vi "Find Class Ancestry.vi"(8 "error in (no error)":errorcluster, 11 "reference in":refnum<vi>) -> (0 "error out":errorcluster, 3 "Class Ancestry":path[](array[path]))   [LabVIEW 2020, in "Test Suite Factory.lvclass"]
uses:
  Test Suite Factory.lvclass
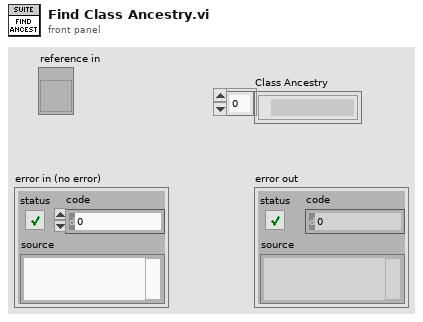
[diagram p1: front panel]
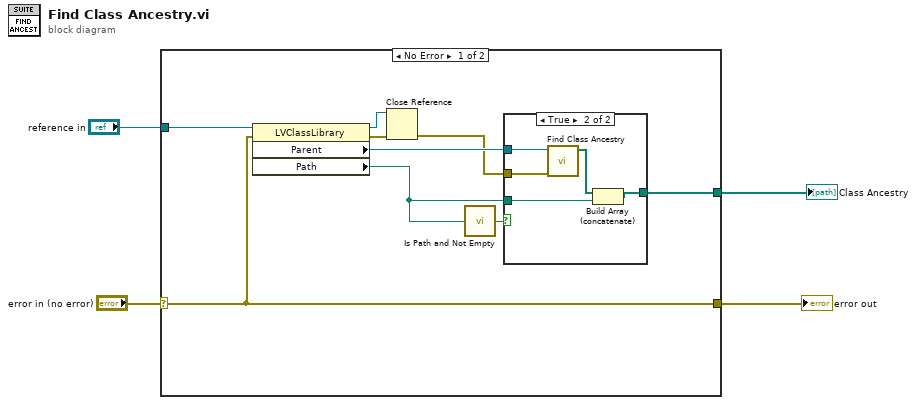
[diagram p0: block diagram]
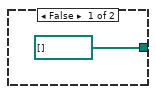
[diagram p2: hidden frame]
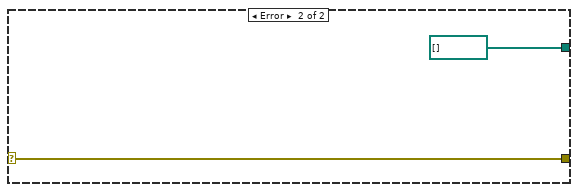
[diagram p3: hidden frame]
diagram:
  n1 = case shown="No Error" "error in (no error)" {
    selector: "error in (no error)" -> [w5 w21]
    tunnel: "reference in" -> [w13 _]
    tunnel: [w11 path[] [] ("Class Ancestry")] -> w3
    tunnel: [w5 w21] -> w1
    frame No Error {
      n2 = property class="LVClassLibrary"(reference=w13, error in=w5) -> (reference out=w9:refnum<vi>, error out=w10:errorcluster, "Parent"=w12:refnum<vi>, "Path"=w7:path)
      n3 = Close Reference(reference=w9, error in (no error)=w10) -> (error out=w8:errorcluster)
      n4 = call <vilib>:"Is Path and Not Empty.vi"("path"=w7) -> ("Is Path and Not Empty?"=w6:bool)  [unwired: 4 in]
      n5 = case shown="True" w6 {
        tunnel: [path[] [] ("Class Ancestry") w17] -> w11
        tunnel: w12 -> [_ w19]
        tunnel: w7 -> [_ w16]
        tunnel: w8 -> [_ w15]
        frame False {
        }
        frame True {
          n6 = call "Find Class Ancestry.vi"("error in (no error)"=w15, "reference in"=w19) -> ("Class Ancestry"=w18:path[])  [unwired: 8 in, 1 out]
          n7 = Build Array (concatenate)(w18, w16) -> (w17:path[])
        }
      }
    }
    frame Error {
    }
  }
  "Class Ancestry" <- w3
  "error out" <- w1
